vi "Get Cell Position.vi"(11 "listbox in":refnum<class "listbox.lvclass">) -> (2 "Cell Position":T1, 3 "listbox out":refnum<class "listbox.lvclass">)   [LabVIEW 2016, in "listbox.lvclass"]
uses:
  listbox.lvclass
  <vilib>/Utility/miscctls.llb/LVRowAndColumnTypeDef.ctl
  listbox.lvclass/listbox.ctl
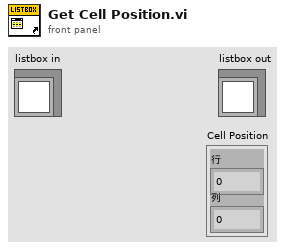
[diagram p1: front panel]
types:
  T1 = typedef "LVRowAndColumnTypeDef.ctl" = cluster{"Row":i32, "Column":i32}
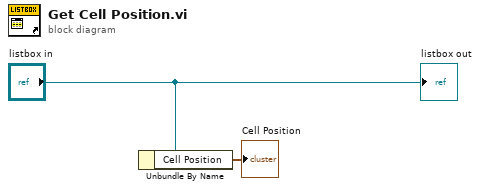
[diagram p0: block diagram]
diagram:
  n1 = Unbundle By Name("listbox in") -> ("Cell Position"=→"Cell Position":T1)
  "listbox out" <- "listbox in"
